vi "Custom Device Offline Path.vi"() -> ()   [LabVIEW 2019, in "Custom Device API.lvlib"]
uses:
  Custom Device API.lvlib
panel:
  in  "Offline Path":path=path "NI VeriStand/Custom Device Offline API"
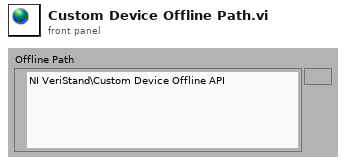
[diagram p1: front panel]
diagram:
